vi "initMightex.vi"() -> (0 "error out":errorcluster)   [LabVIEW 2016]
uses:
  lib/SSClassic_USBCamera_SDK.dll
panel:
  out "ModuleNo:":string
  out "SerialNo:":string
  out "OK to run":bool
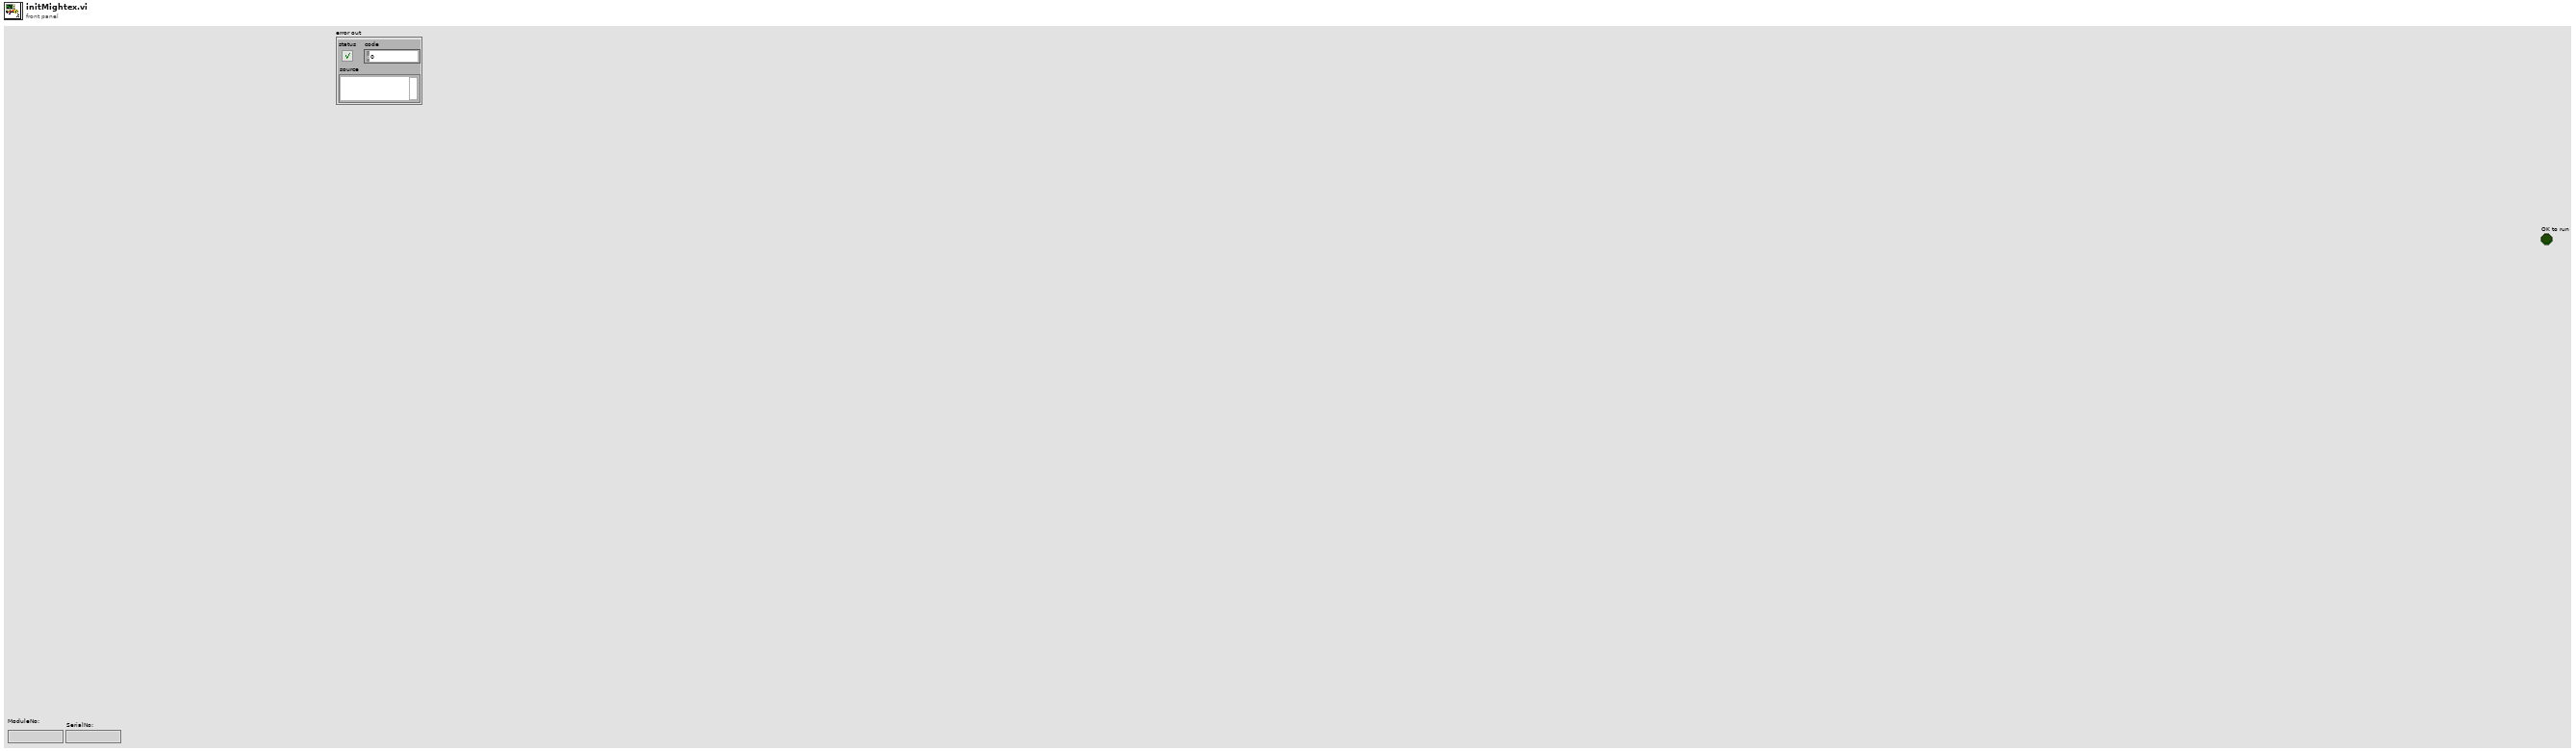
[diagram p1: front panel]
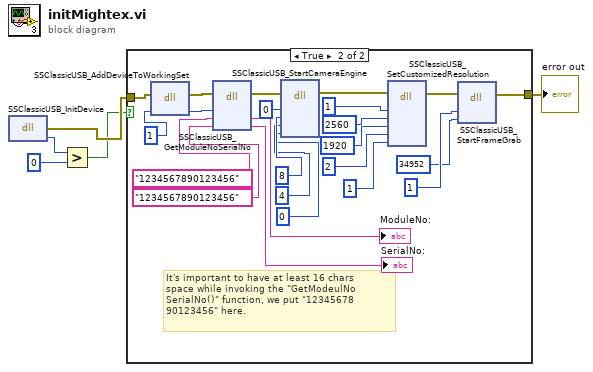
[diagram p0: block diagram]
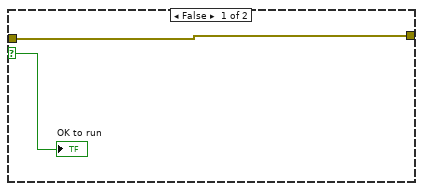
[diagram p2: hidden frame]
diagram:
  n1 = dll-call lib="D:/All users/PoSheng/src/lib/SSClassic_USBCamera_SDK.dll" fn="SSClassicUSB_InitDevice" ("CCD_USBCamera_SDK.dll:CCDUSB_InitDevice")() -> (error out=w3:errorcluster, "ReturnValue"=w5:u32)  [unwired: 3 in, 1 out]
  n2 = Greater?(x=w5, y=0) -> (0:w2:bool)
  n3 = case shown="True" w2 {
    selector: w2 -> [w7 _]
    tunnel: w3 -> [w6 w30]
    tunnel: [w6 w23] -> w1
    frame False {
      "OK to run" <- w7
    }
    frame True {
      # "It's important to have at least 16 chars\nspace while invoking the \"GetModeulNo\nSerialNo()\" function, we put \"12345678\n90123456\" here."
      n4 = dll-call lib="D:/All users/PoSheng/src/lib/SSClassic_USBCamera_SDK.dll" fn="SSClassicUSB_AddDeviceToWorkingSet" ("CCD_USBCamera_SDK.dll:CCDUSB_AddDeviceToWorkingSet")(error in=w30, "Arg1"=1) -> (error out=w29:errorcluster, "Arg1"=w27:i32)  [unwired: 3 in, 1 out]
      n5 = dll-call lib="D:/All users/PoSheng/src/lib/SSClassic_USBCamera_SDK.dll" fn="SSClassicUSB_GetModuleNoSerialNo" ("CCD_USBCamera_SDK.dll:CCDUSB_GetModuleNoSerialNo")(error in=w29, "Arg1"=w27, "Arg2"="1234567890123456", "Arg3"="1234567890123456") -> (error out=w25:errorcluster, "Arg2"=→"ModuleNo:":string, "Arg3"=→"SerialNo:":string)  [unwired: 4 in, 1 out]
      n6 = dll-call lib="D:/All users/PoSheng/src/lib/SSClassic_USBCamera_SDK.dll" fn="SSClassicUSB_StartCameraEngine" ("CCD_USBCamera_SDK.dll:CCDUSB_StartCameraEngine")(error in=w25, "Arg1"=0, "Arg2"=8, "Arg3"=4, "Arg4"=0) -> (error out=w18:errorcluster)  [unwired: 7 in, 1 out]
      n7 = dll-call lib="D:/All users/PoSheng/src/lib/SSClassic_USBCamera_SDK.dll" fn="SSClassicUSB_SetCustomizedResolution" ("BUF_USBCamera_SDK.dll:BUFUSB_SetCustomizedResolution")(error in=w18, "Arg1"=1, "Arg2"=2560, "Arg3"=1920, "Arg4"=2, "Arg5"=u32 1) -> (error out=w17:errorcluster)  [unwired: 8 in, 1 out]
      n8 = dll-call lib="D:/All users/PoSheng/src/lib/SSClassic_USBCamera_SDK.dll" fn="SSClassicUSB_StartFrameGrab" ("CCD_USBCamera_SDK.dll:CCDUSB_StartFrameGrab")(error in=w17, "Arg1"=1, "Arg2"=34952) -> (error out=w23:errorcluster)  [unwired: 5 in, 1 out]
    }
  }
  "error out" <- w1
